vi "CliGetCpuInfo.vi"(0 "ref in":u64, 11 "error in (no error)":errorcluster) -> (1 "ModuleTypeName":string, 2 "SerialNumber":string, 3 "ASName":string, 4 "ref out":u64, 6 "Result":i32, 13 "ModuleName":string, 14 "Copyright":string, 15 "error out":errorcluster)   [LabVIEW 2016, in "Snap7.lvlib"]
uses:
  Snap7.lvlib
  win32/lv_snap7.dll
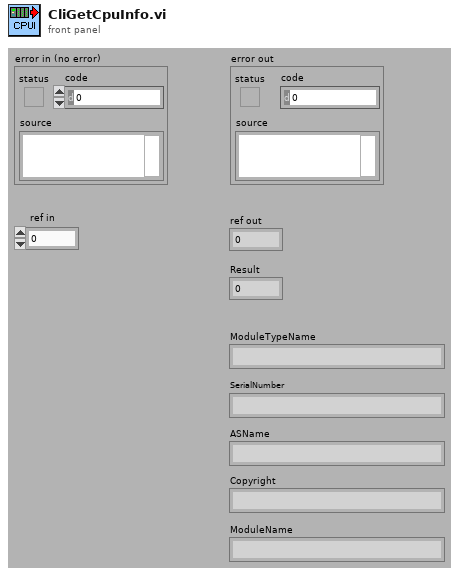
[diagram p1: front panel]
types:
  T1 = enum16{"big-endian, network order", "native, host order", "little-endian"}
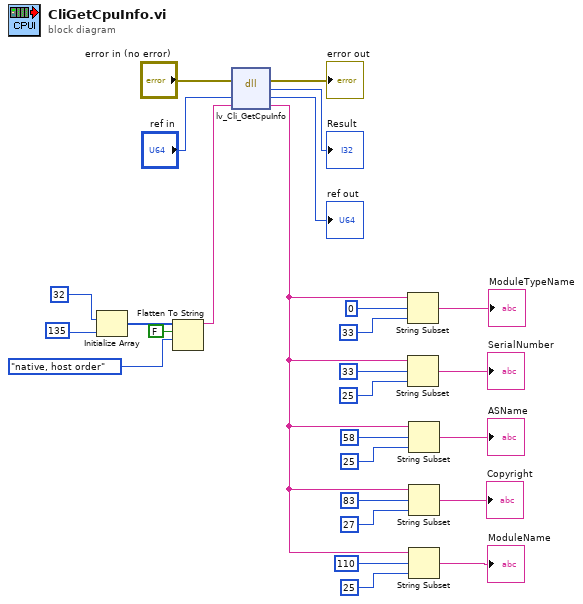
[diagram p0: block diagram]
diagram:
  n1 = Initialize Array(u8 32, 135) -> (w1:u8[])
  n2 = Flatten To String(anything=w1, prepend array or string size? (T)=FALSE, byte order (0:big-endian, network order)=T1."native, host order") -> (data string=w18:string)  [unwired: 1 in, 2 out]
  n3 = dll-call lib="D:/maszup/svn/LineTraceSystem/SOFTWARE/sources/Drivers/PLC/Snap7/lib/win32/lv_snap7.dll" fn="lv_Cli_GetCpuInfo"(error in="error in (no error)", "Client"="ref in", "var_Info"=w18) -> (error out=→"error out":errorcluster, "return type"=→"Result":i32, "Client"=→"ref out":u64, "var_Info"=w2:string)  [unwired: 2 in, 1 out]
  n4 = String Subset(string=w2, offset (0)=0, length (rest)=33 ("length (rest)")) -> (substring=→"ModuleTypeName":string)
  n5 = String Subset(string=w2, offset (0)=33, length (rest)=25 ("length (rest)")) -> (substring=→"SerialNumber":string)
  n6 = String Subset(string=w2, offset (0)=58, length (rest)=25 ("length (rest)")) -> (substring=→"ASName":string)
  n7 = String Subset(string=w2, offset (0)=83, length (rest)=27 ("length (rest)")) -> (substring=→"Copyright":string)
  n8 = String Subset(string=w2, offset (0)=110, length (rest)=25 ("length (rest)")) -> (substring=→"ModuleName":string)
